vi "abouttest.vi"   [LabVIEW 2015]
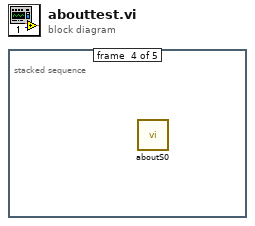
[diagram p0: block diagram]
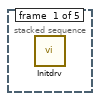
[diagram p2: hidden frame]
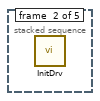
[diagram p3: hidden frame]
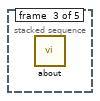
[diagram p4: hidden frame]
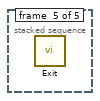
[diagram p5: hidden frame]
diagram:
  n1 = stacked-sequence {
    frame #0 {
      n2 = call "Initdrv.vi"() -> ()  [unwired: 1 in]
    }
    frame #1 {
      n3 = call "InitDrv.vi"() -> ()  [unwired: 1 in]
    }
    frame #2 {
      n4 = call "about.vi"() -> ()  [unwired: 1 in]
    }
    frame #3 {
      n5 = call "aboutS0.vi"() -> ()  [unwired: 1 in]
    }
    frame #4 {
      n6 = call "Exit.vi"() -> ()  [unwired: 1 in]
    }
  }
